vi "Stage Reference Follower v1.3.vi"(6 "stop":bool, 8 "Stage PID Cluster":T1={"Stage Z PID"={"Kp"=0.0005, "Kd"=0.001, "Ki"=0.0}, "Stage Y PID"={"Kp"=0.0003, "Kd"=0.01, "Ki"=0.0}, "Stage X PID"={"Kp"=0.0003, "Kd"=0.01, "Ki"=0.0}}, 9 "Stage cmd Posit [mm]":dbl[](array[numeric])=[6.0, 6.0, 6.0], 10 "error in":errorcluster, 11 "FPGA VI Reference In":refnum<k20>) -> (1 "Stage out Posit [mm]":dbl[](array[numeric])=[12.0, 0.0, 0.0], 2 "error out":errorcluster, 3 "FPGA VI Reference Out":refnum<k20>)   [LabVIEW 2010]
uses:
  <vilib>/rvi/interface/nirviReadWriteControl/nirviReadWriteControl.xnode
  Library/jmslib.lvlib
  FPGA Bitfiles/IRISSControl_FPGATarget_IRISSFPGAIOv3.3_r-h2UkgnQFc.lvbitx
  IRISS_FPGA_IO_v3.3.vi
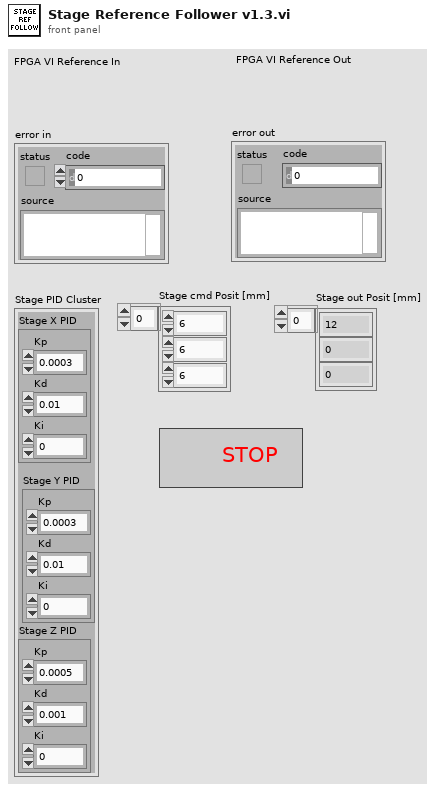
[diagram p1: front panel]
types:
  T1 = cluster{"Stage Z PID":cluster{"Kp":dbl, "Kd":dbl, "Ki":dbl}, "Stage Y PID":cluster{"Kp":dbl, "Kd":dbl, "Ki":dbl}, "Stage X PID":cluster{"Kp":dbl, "Kd":dbl, "Ki":dbl}}
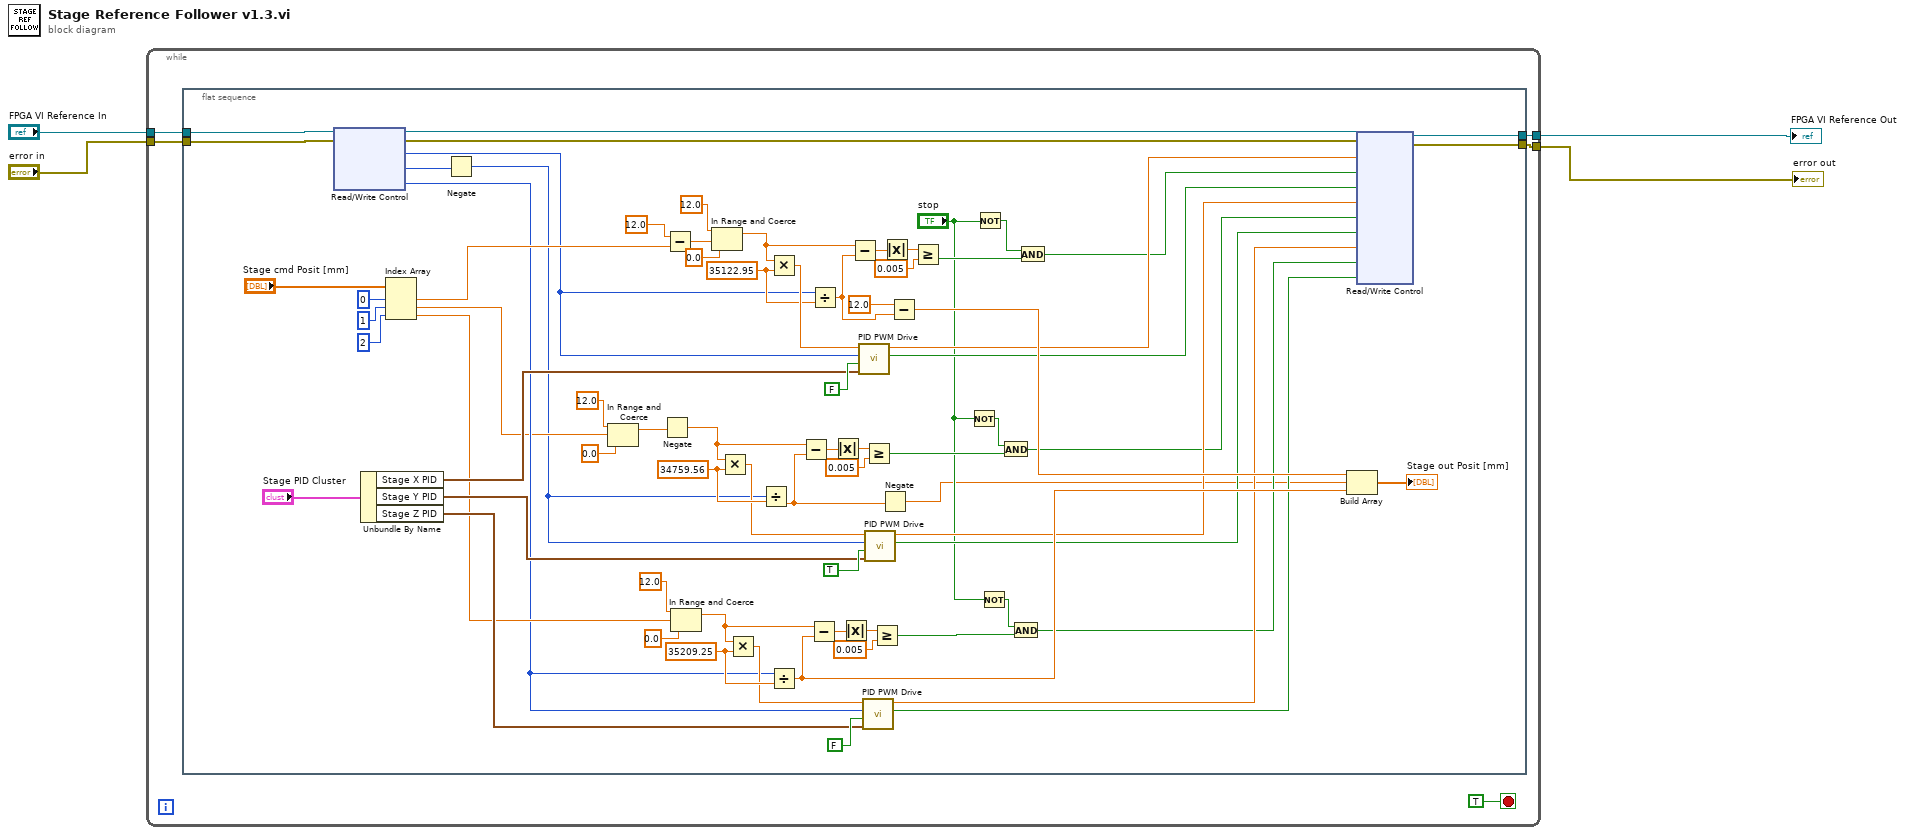
[diagram p0: block diagram]
diagram:
  n1 = while {
    tunnel: "FPGA VI Reference In" -> [w9]
    tunnel: "error in" -> [w8]
    tunnel: [w7] -> w4
    tunnel: [w6] -> w3
    stop <- TRUE stop-if-true
    n2 = flat-sequence {
      tunnel: w9 -> [w83]
      tunnel: w8 -> [w82]
      tunnel: [w22] -> w7
      tunnel: [w21] -> w6
      frame #0 {
        w49 = 35209.25 ("y")
        w63 = 34759.56 ("y")
        w78 = 35122.95 ("y")
        n3 = xnode "Read/Write Control"("FPGA VI Reference In"=w83, "error in"=w82) -> ("FPGA VI Reference Out"=w24:refnum<k20>, "error out"=w23:errorcluster, "Position X"=w31:i32, "Position Y"=w13:i32, "Position Z"=w20:i32)
        n4 = Unbundle By Name("Stage PID Cluster") -> ("Stage X PID"=w56:cluster{"Kp":dbl, "Kd":dbl, "Ki":dbl}, "Stage Y PID"=w55:cluster{"Kp":dbl, "Kd":dbl, "Ki":dbl}, "Stage Z PID"=w43:cluster{"Kp":dbl, "Kd":dbl, "Ki":dbl})
        n5 = Index Array(array="Stage cmd Posit [mm]", index #1=0 ("index"), index #2=1 ("index"), index #3=2 ("index")) -> (element #1=w68:dbl, element #2=w16:dbl, element #3=w39:dbl)
        n6 = Negate(x=w13) -> (-x=w12:i32)
        n7 = In Range and Coerce(upper limit=12.0, x=w16, lower limit=0.0) -> (coerced(x)=w15:dbl)  [unwired: 1 out]
        n8 = Negate(x=w15) -> (-x=w14:dbl)
        n9 = Subtract(x=12.0 ("upper limit"), y=w68) -> (x-y=w72:dbl)
        n10 = In Range and Coerce(upper limit=12.0, x=w39, lower limit=0.0) -> (coerced(x)=w51:dbl)  [unwired: 1 out]
        n11 = In Range and Coerce(upper limit=12.0, x=w72, lower limit=0.0) -> (coerced(x)=w76:dbl)  [unwired: 1 out]
        n12 = Multiply(x=w14, y=w63) -> (x*y=w61:dbl)
        n13 = Multiply(x=w51, y=w49) -> (x*y=w47:dbl)
        n14 = Divide(x=w12, y=w63) -> (x/y=w11:dbl)
        n15 = Multiply(x=w76, y=w78) -> (x*y=w80:dbl)
        n16 = Divide(x=w20, y=w49) -> (x/y=w35:dbl)
        n17 = Subtract(x=w14, y=w11) -> (x-y=w65:dbl)
        n18 = Subtract(x=w51, y=w35) -> (x-y=w52:dbl)
        n19 = Divide(x=w31, y=w78) -> (x/y=w70:dbl)
        n20 = Absolute Value(x=w65) -> (abs(x)=w66:dbl)
        n21 = Absolute Value(x=w52) -> (abs(x)=w53:dbl)
        n22 = Subtract(x=w76, y=w70) -> (x-y=w75:dbl)
        n23 = call "PID PWM Drive.vi"("PID Gains"=w56, "Reverse Motor?"=FALSE, "Encoder Position"=w31, "Reference"=w80) -> ("Direction"=w30:bool, "Duty Cycle"=w33:dbl)  [unwired: 5 in, 1 out]
        n24 = call "PID PWM Drive.vi"("PID Gains"=w43, "Reverse Motor?"=FALSE, "Encoder Position"=w20, "Reference"=w47) -> ("Direction"=w25:bool, "Duty Cycle"=w27:dbl)  [unwired: 5 in, 1 out]
        n25 = Greater Or Equal?(x=w66, y=0.005) -> (x >= y?=w59:bool)
        n26 = call "PID PWM Drive.vi"("PID Gains"=w55, "Reverse Motor?"=TRUE, "Encoder Position"=w12, "Reference"=w61) -> ("Direction"=w28:bool, "Duty Cycle"=w32:dbl)  [unwired: 5 in, 1 out]
        n27 = Greater Or Equal?(x=w53, y=0.005) -> (x >= y?=w45:bool)
        n28 = Negate(x=w11) -> (-x=w10:dbl)
        n29 = Absolute Value(x=w75) -> (abs(x)=w74:dbl)
        n30 = Subtract(x=12.0 ("upper limit"), y=w70) -> (x-y=w36:dbl)
        n31 = Greater Or Equal?(x=w74, y=0.005) -> (x >= y?=w38:bool)
        n32 = Not(x="stop") -> (.not. x?=w58:bool)
        n33 = Not(x="stop") -> (.not. x?=w37:bool)
        n34 = Not(x="stop") -> (.not. x?=w44:bool)
        n35 = And(x=w58, y=w59) -> (x .and. y?=w29:bool)
        n36 = And(x=w44, y=w45) -> (x .and. y?=w26:bool)
        n37 = And(x=w37, y=w38) -> (x .and. y?=w19:bool)
        n38 = Build Array(w36, w10, w35) -> (→"Stage out Posit [mm]":dbl[])
        n39 = xnode "Read/Write Control"("FPGA VI Reference In"=w24, "error in"=w23, "X DC"=w33, "INHB X"=w19, "DIR X"=w30, "Y DC"=w32, "INHB Y"=w29, "DIR Y"=w28, "Z DC"=w27, "INHB Z"=w26, "DIR Z"=w25) -> ("FPGA VI Reference Out"=w22:refnum<k20>, "error out"=w21:errorcluster)
      }
    }
  }
  "error out" <- w3
  "FPGA VI Reference Out" <- w4
